vi "open and verify serial port.vi"(0 "VISA resource name":refnum<visa-resource-name>, 11 "error in (no error)":errorcluster) -> (4 "VISA resource name out":refnum<visa-resource-name>, 6 "port opened":bool, 8 "version":dbl, 10 "message":string, 15 "error out":errorcluster)   [LabVIEW 2017]
uses:
  <vilib>/Instr/_visa.llb/VISA Set IO Buffer Mask.ctl
  typedefs/commandType.ctl
  <vilib>/Instr/_visa.llb/VISA Flush IO Buffer Mask.ctl
  <vilib>/Instr/_visa.llb/VISA Configure Serial Port (Instr).vi
  <vilib>/Utility/error.llb/DialogType.ctl
panel:
  out "command string 3":string
  out "command string 2":string
  out "command string":string
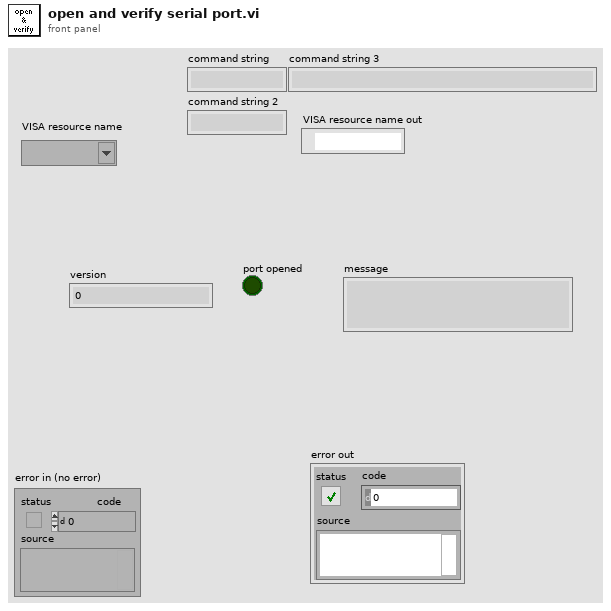
[diagram p1: front panel]
types:
  T1 = typedef "commandType.ctl" = enum16{"G - set gain", "C - activate coil", "D - deactivate coil", "L - set LED", "A - set AUTO", "V - set verbose", "T - set transmission", "R - get version", "Z - zero accelerometer", "F - set auto-flash led", "S - synchronize serial"}
  T2 = typedef "VISA Flush IO Buffer Mask.ctl" = u16
  T3 = typedef "VISA Set IO Buffer Mask.ctl" = u16
  T4 = typedef "DialogType.ctl" = u16
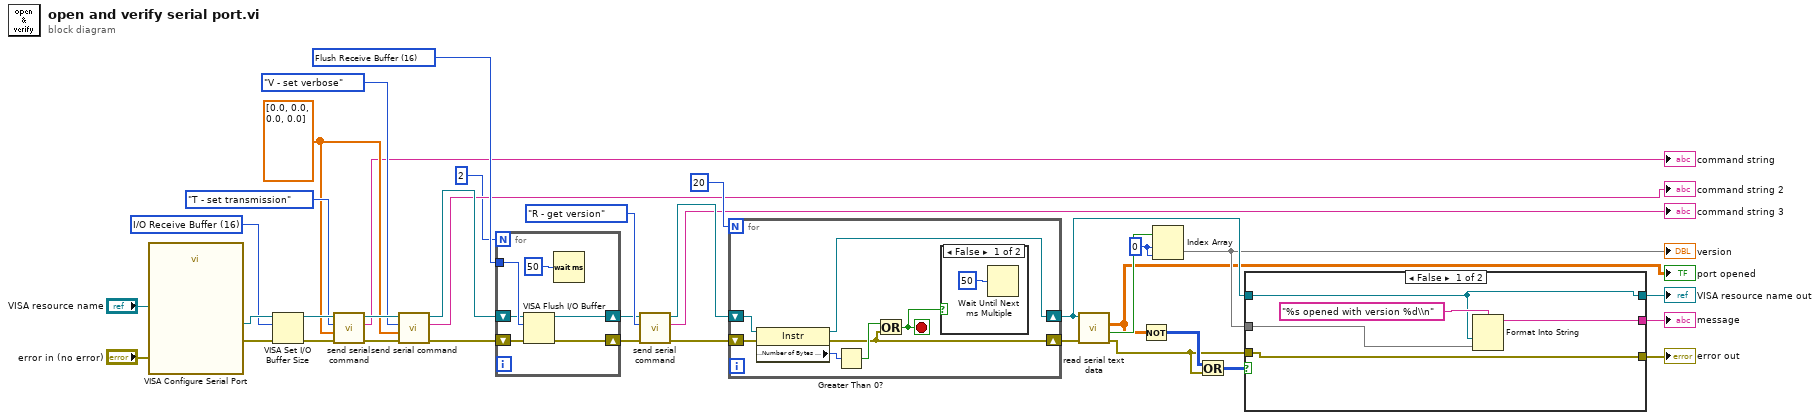
[diagram p0: block diagram]
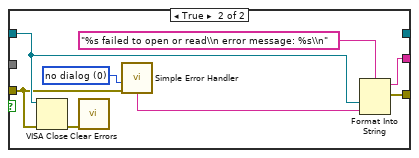
[diagram p2: hidden frame]
diagram:
  w16 = 0 ("index (row)")
  w18 = dbl[] [0.0, 0.0, 0.0, 0.0]
  w28 = T2 16 items=["Flush Receive Buffer"=16, "Write Transmit Buffer to Device"=32, "Flush Receive Buffer (No I/O)"=64, "Flush Transmit Buffer"=128] ("Mask")
  w35 = T3 16 items=["I/O Receive Buffer"=16, "I/O Transmit Buffer"=32, "I/O Receive and Transmit Buffer"=48] ("Mask")
  n1 = call-poly "VISA Configure Serial Port"("VISA resource name"="VISA resource name", "error in (no error)"="error in (no error)") -> ("VISA resource name out"=w37:refnum<visa-resource-name>, "error out"=w34:errorcluster)  [unwired: 12 in]
  n2 = VISA Set I/O Buffer Size(VISA resource name=w37, mask (16)=w35, error in (no error)=w34) -> (VISA resource name out=w25:refnum<visa-resource-name>, error out=w26:errorcluster)  [unwired: 1 in]
  n3 = call "send serial command.vi"("error in (no error)"=w26, "data"=w18, "Command"=commandType."T - set transmission", "visa resource"=w25) -> ("error out"=w23:errorcluster, "command string"=→"command string":string, "VISA resource name out"=w20:refnum<visa-resource-name>)  [unwired: 5 in]
  n4 = call "send serial command.vi"("error in (no error)"=w23, "data"=w18, "Command"=commandType."V - set verbose", "visa resource"=w20) -> ("error out"=w22:errorcluster, "command string"=→"command string 2":string, "VISA resource name out"=w21:refnum<visa-resource-name>)  [unwired: 5 in]
  n5 = for {
    N: 2 -> [_]
    tunnel: w28 -> [w41]
    shift-right: [w42] -> w29
    shift-left: w22 -> [w40]
    shift-right: [w43] -> w30
    shift-left: w21 -> [w39]
    n6 = VISA Flush I/O Buffer(VISA resource name=w39, mask (16)=w41, error in (no error)=w40) -> (VISA resource name out=w43:refnum<visa-resource-name>, error out=w42:errorcluster)
    n7 = Wait (ms)(milliseconds to wait=u32 50) -> ()  [unwired: 1 out]
  }
  n8 = call "send serial command.vi"("error in (no error)"=w29, "Command"=commandType."R - get version", "visa resource"=w30) -> ("error out"=w32:errorcluster, "command string"=→"command string 3":string, "VISA resource name out"=w31:refnum<visa-resource-name>)  [unwired: 6 in]
  n9 = for {
    N: 20 -> [_]
    shift-right: [w46] -> w27
    shift-left: w32 -> [w49]
    shift-right: [w45] -> w12
    shift-left: w31 -> [w50]
    stop <- w44 stop-if-true
    n10 = property class="Instr"(reference=w50, error in=w49) -> (reference out=w45:refnum<visa-resource-name>, error out=w46:errorcluster, "Serial Settings:Number of Bytes at Serial Port"=w48:u32)
    n11 = Greater Than 0?(x=w48) -> (x > 0?=w47:bool)
    n12 = Or(x=w47, y=w46) -> (x .or. y?=w44:bool)
    n13 = case shown="False" w44 {
      frame False {
        n14 = Wait Until Next ms Multiple(millisecond multiple=u32 50) -> ()  [unwired: 1 out]
      }
      frame True {
      }
    }
  }
  n15 = call "read serial text data.vi"("error in (no error)"=w27, "serial port"=w12) -> ("error out"=w11:errorcluster, "data read"=w17:bool, "serial data"=w2:dbl[][])  [unwired: 6 in, 1 out]
  "port opened" <- w2
  n16 = Not(x=w2) -> (.not. x?=w14:u32[][])
  n17 = Index Array(array=w17, index (row)=w16, index (col)=w16) -> (element=w10)
  "version" <- w10
  n18 = Or(x=w14, y=w11) -> (x .or. y?=w13:u32[][])
  n19 = case shown="False" w13 {
    tunnel: w12 -> [w54 w63]
    tunnel: w11 -> [w56 w62]
    tunnel: [w54 _] -> w7
    tunnel: [w56 w59] -> w8
    tunnel: w10 -> [w53 _]
    tunnel: [w52 w58] -> w9
    frame False {
      n20 = Format Into String(format string="%s opened with version %d\\n", w54, w53) -> (resulting string=w52:string)  [unwired: 2 in, 1 out]
    }
    frame True {
      w61 = T4 0 items=["no dialog", "OK message", "continue or stop message", "OK message + warnings", "continue/stop + warnings"] ("type of dialog (OK msg:1)")
      n21 = VISA Close(VISA resource name=w63, error in (no error)=w62) -> (error out=w57:errorcluster)
      n22 = call <vilib>:"Clear Errors.vi"("error in (no error)"=w57) -> ()  [unwired: 5 in, 2 out]
      n23 = call <vilib>:"Simple Error Handler.vi"("type of dialog (OK msg:1)"=w61, "error in (no error)"=w62) -> ("message"=w60:string)  [unwired: 3 in, 4 out]
      n24 = Format Into String(format string="%s failed to open or read\\n error message: %s\\n", w63, w60) -> (resulting string=w58:string, error out=w59:errorcluster)  [unwired: 2 in]
    }
  }
  "message" <- w9
  "error out" <- w8
  "VISA resource name out" <- w7
